vi "SubPanel_DataCollection_Rev11_v7.vi"(0 "DCPowerInformationClusterArray_Input":T2(array[cluster]), 1 "VISAPowerInfoInputArray":T7(array[cluster]), 2 "Run Data SubPanel Input":T6, 3 "RF Block Parameters":T5, 4 "Oscilloscope Info Array":T4(array[cluster]) {"vertical coupling" items=["AC", "DC", "Ground"]}, 6 "New Run?":bool, 7 "error in":errorcluster) -> (16 "data going into the binary file":T1, 20 "DCPowerInformationClusterArray_Output":T2(array[cluster]), 21 "VISAPowerInfoInputOutput":T7(array[cluster]), 22 "Run Data SubPanel Output":T6, 23 "RF Block Parameters Output":T5, 24 "Oscilloscope Info Array Output":T4(array[cluster]) {"vertical coupling" items=["AC", "DC", "Ground"]}, 25 "Reinitialize?":bool, 26 "Data Was Collected?":bool, 27 "error out":errorcluster)   [LabVIEW 2019]
uses:
  Controls/QueueDataControl.ctl
  Controls/DataBlockControl.ctl
  Controls/QueueDataControl_V2.ctl
  <vilib>/Analysis/NI_AALBase.lvlib
  Controls/QueueDataControl_V3.ctl
  <vilib>/Analysis/1siggen.llb/Ramp Pattern by Delta.vi
  <vilib>/Utility/file.llb/Write Delimited Spreadsheet (string).vi
  Controls/RFBlockControl.ctl
  <instrlib>/niScope/Controls/niScope vertical coupling.ctl
panel:
  out "Current 3":waveform(dbl)[](graph)
  out "Voltage 3":waveform(dbl)[](graph)
  out "DCPowerInfoArray":string[][](array[string])
  out "Array":string[][][](array[string])
  out "Current Measurements":cluster{dbl[], dbl[]}[](graph)
  out "Voltage Measurements":cluster{dbl[], dbl[]}[](graph)
  out "DCPowerInformationClusterArray_Input 2":T2(array[cluster])
  out "Exiting":bool
  out "Full Run Information":string
  out "Ready For Next Run?":bool
  in  "Next Run":bool
  out "Latchup Output Data":dbl[][](array[numeric])
  out "Recording Data":bool
  out "Current 2":waveform(dbl)[](graph)
  out "Voltage 2":waveform(dbl)[](graph)
  out "Current":waveform(dbl)[](graph)
  out "Voltage":waveform(dbl)[](graph)
  in  "End Collecting":bool
  in  "Record Data Toggle":bool
  out "error of collection":errorcluster
  in  "force exit SubVI":bool
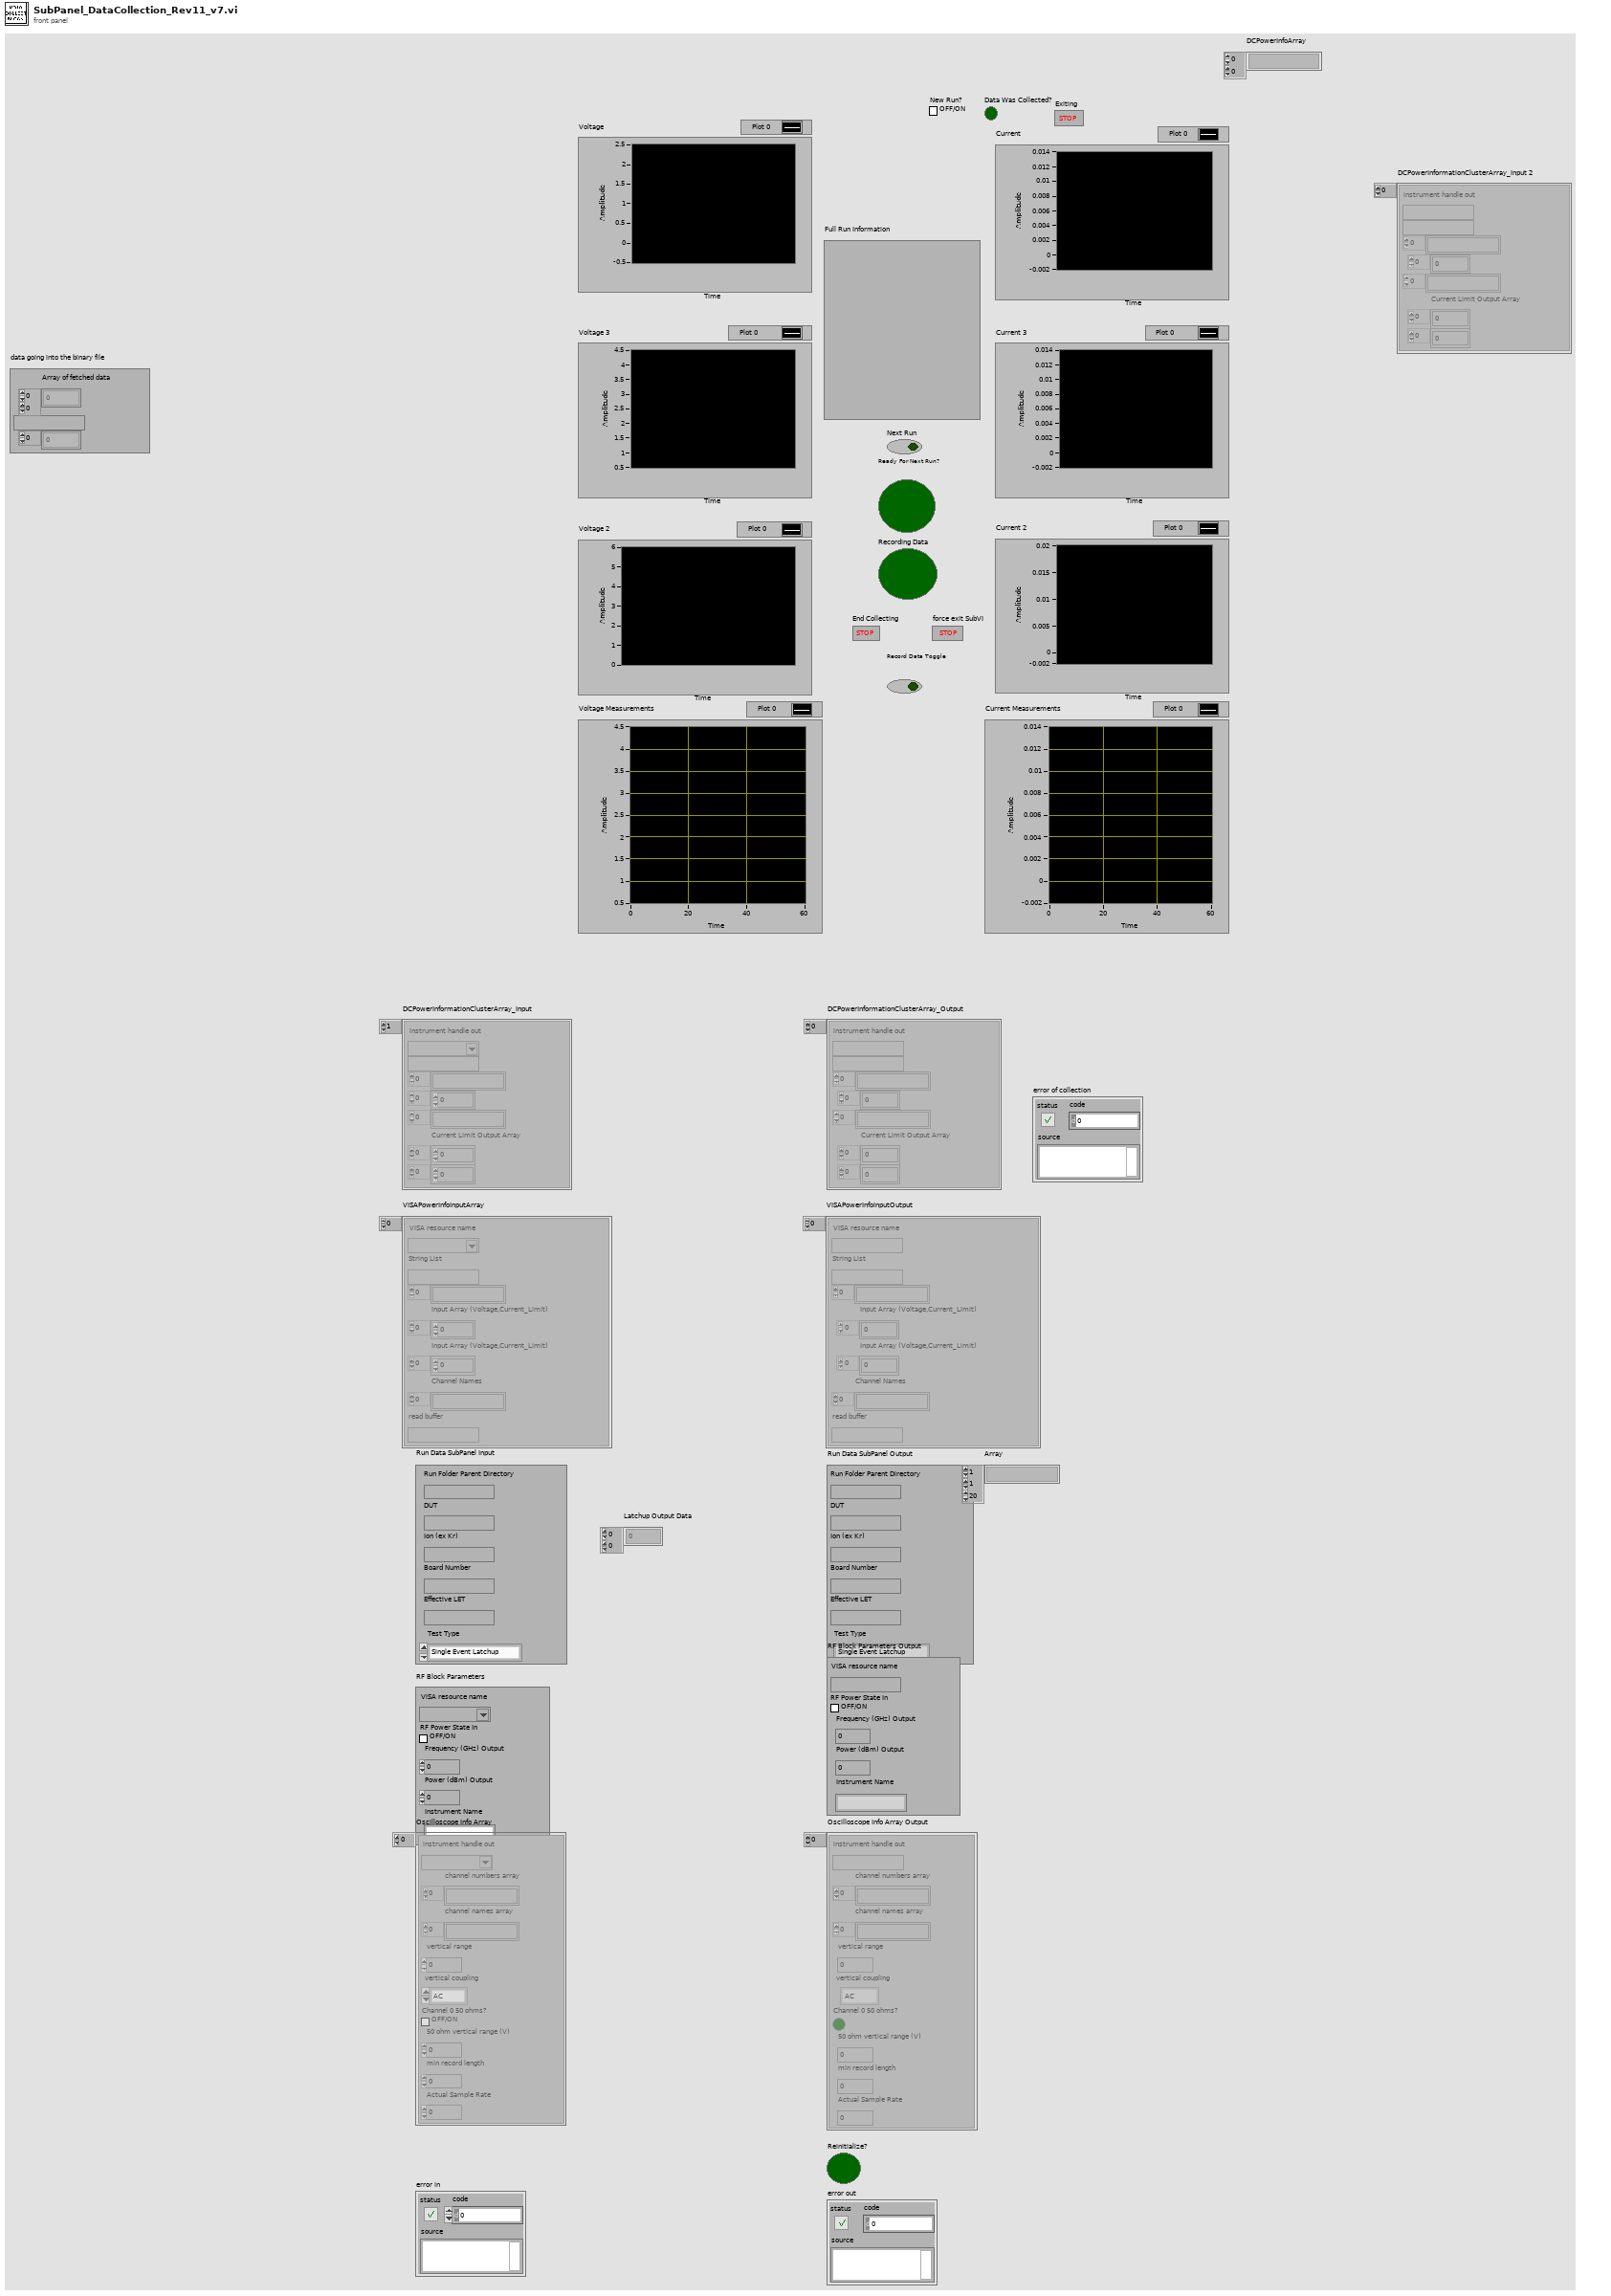
[diagram p1: front panel]
types:
  T1 = cluster{"Array of fetched data":dbl[][], string, i32[]}
  T2 = cluster{"instrument handle out":refnum<k15>, string, string[], dbl[], string[], "Current Limit Output Array":dbl[], dbl[]}[]
  T3 = typedef "niScope vertical coupling.ctl" = i32
  T4 = cluster{"instrument handle out":refnum<k15>, "channel numbers array":string[], "channel names array":string[], "vertical range":dbl, "vertical coupling":T3, "Channel 0 50 ohms?":bool, "50 ohm vertical range (V)":dbl, "min record length":i32, "Actual Sample Rate":dbl}[]
  T5 = typedef "RFBlockControl.ctl" = cluster{"VISA resource name":refnum<visa-resource-name>, "RF Power State In":bool, "Frequency (GHz) Output":dbl, "Power (dBm) Output":dbl, "Instrument Name":string}
  T6 = typedef "DataBlockControl.ctl" = cluster{"Run Folder Parent Directory":path, "DUT":string, "Ion (ex Kr)":string, "Board Number":string, "Effective LET":string, "Test Type":enum16{"Single Event Latchup", "Single Event Transient", "Single Event Upset"}}
  T7 = cluster{"VISA resource name":refnum<visa-resource-name>, "String List":string, string[], "Input Array (Voltage,Current_Limit)":dbl[], "Input Array (Voltage,Current_Limit)":dbl[], "Channel Names":string[], "read buffer":string}[]
  T8 = typedef "QueueDataControl_V3.ctl" = cluster{"Array of fetched data":dbl[][][], "Channel Names Array":string[], "Voltage Waveform Array":waveform(dbl)[], "Current Waveform Array":waveform(dbl)[], "Resetting Time":timestamp}
  T9 = typedef "QueueDataControl_V2.ctl" = cluster{"Time Stamp Array":timestamp[], "Initial Time":timestamp, "dt measurement array":dbl[], "samples per capture":i32[], "voltage measurements":dbl[][], "current measurements":dbl[][]}
  T10 = cluster{"IVI Refnum out":refnum<k15>, string, "voltage level channel 23":dbl, "Channel Name 23":string, "Current Limit":dbl, "Measure Record dt":dbl, string}[]
  T11 = cluster{"created path":path, "DCPowerInformation_byChannel":cluster{"IVI Refnum out":refnum<k15>, string, "voltage level channel 23":dbl, "Channel Name 23":string, "Current Limit":dbl, "Measure Record dt":dbl, string}[], string[]}
  T12 = typedef "QueueDataControl.ctl" = cluster{"Rolling Timer":timestamp, "Initial Time":timestamp, "dt between samples":dbl[], "number of samples per fetch":i32[], "voltage measurements":dbl[][], "current measurements":dbl[][]}
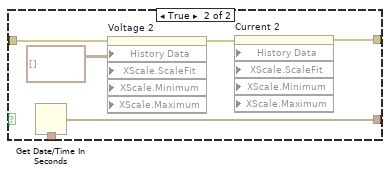
[diagram p2: hidden frame]
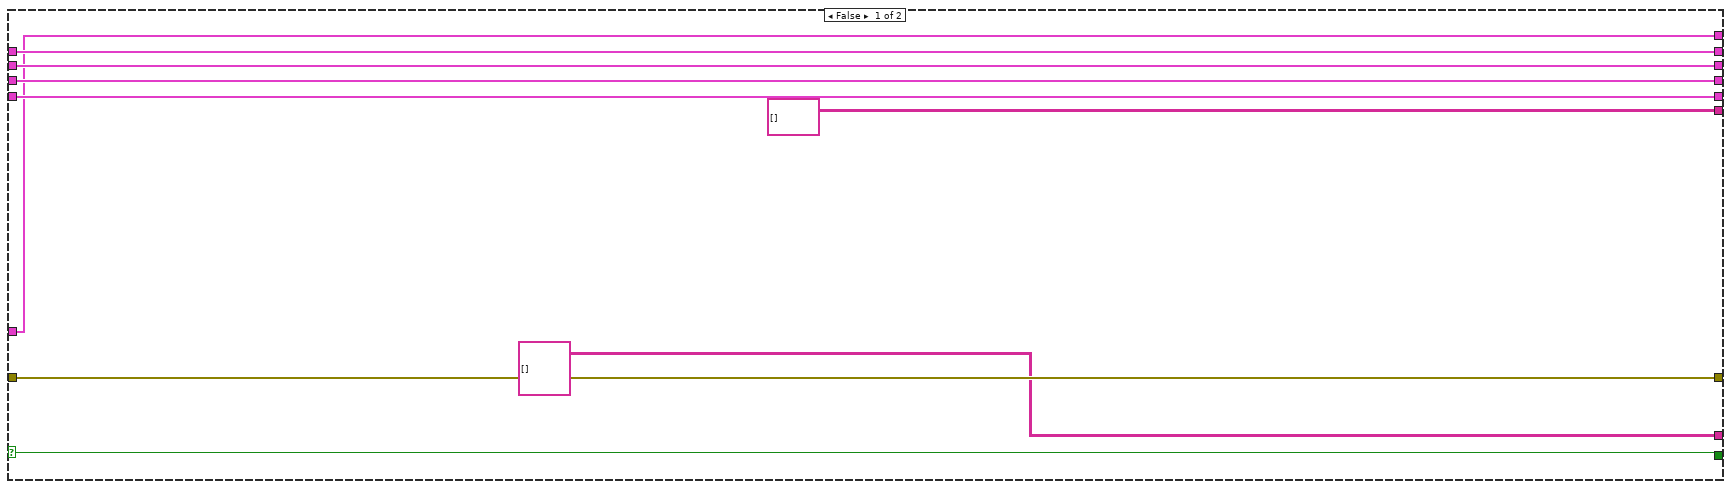
[diagram p4: hidden frame]
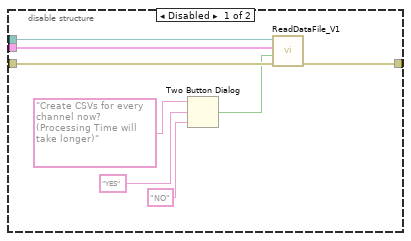
[diagram p5: hidden frame]
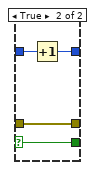
[diagram p6: hidden frame]
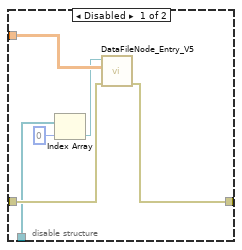
[diagram p9: hidden frame]
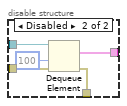
[diagram p10: hidden frame]
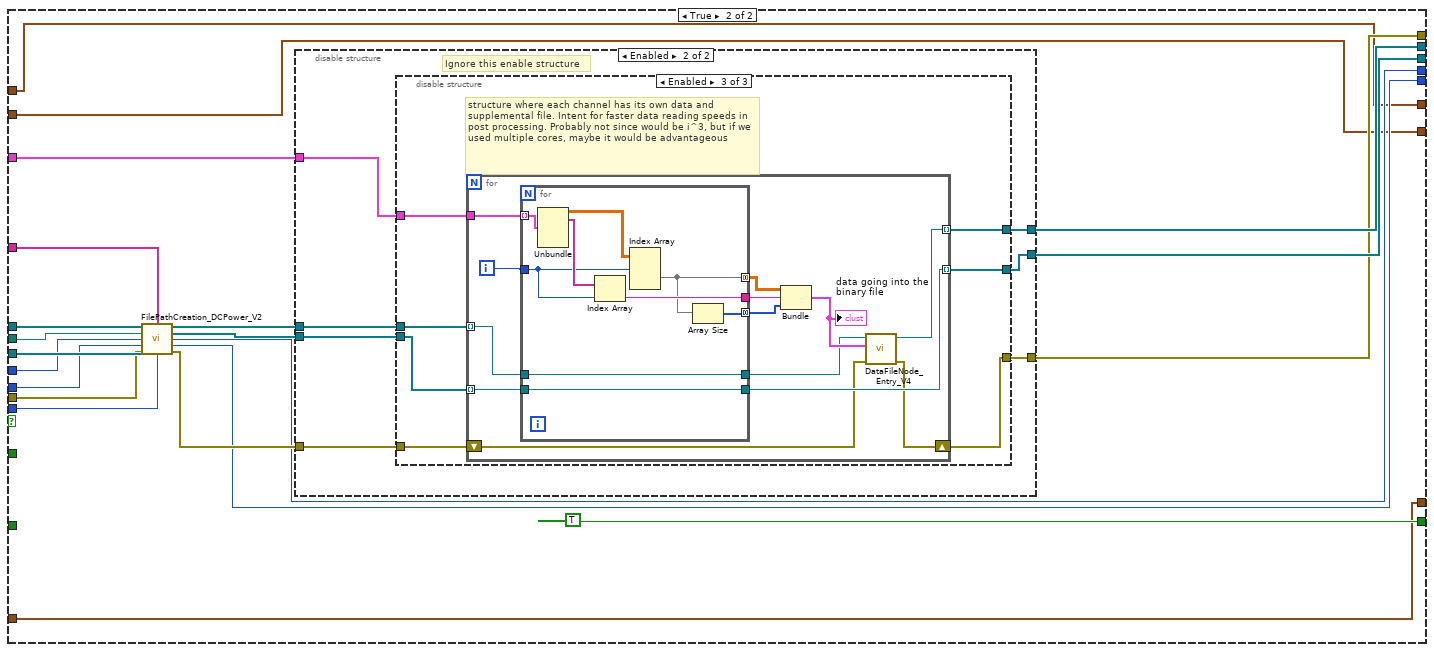
[diagram p13: hidden frame]
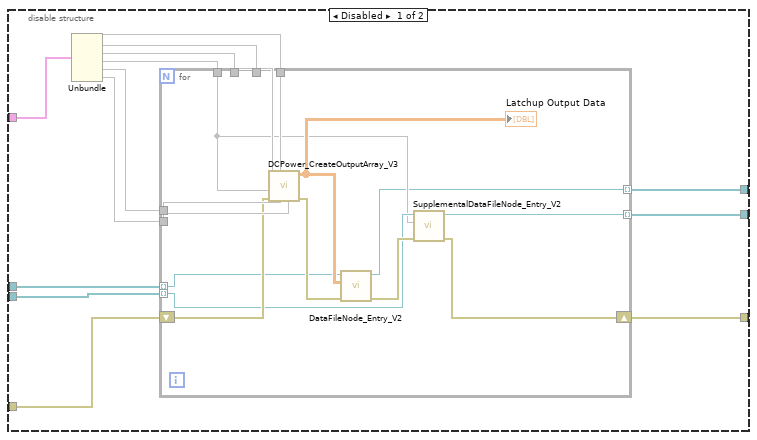
[diagram p14: hidden frame]
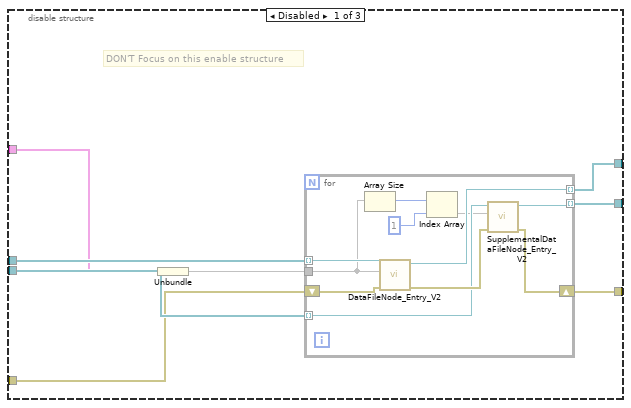
[diagram p15: hidden frame]
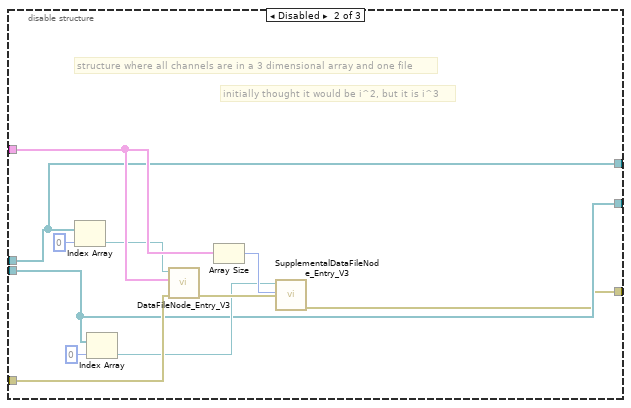
[diagram p16: hidden frame]
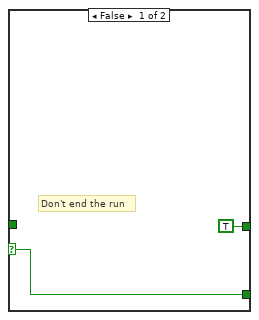
[diagram p18: hidden frame]
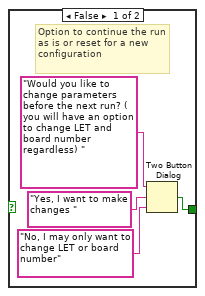
[diagram p19: hidden frame]
diagram:
  (unwired) string[] ["Instrument Name", "Channel Name", "Instrument Channel Number", "Voltage (V)", "Current Limit (A)", "Measure Record delta Time (s)"] ("new element/subarray")
  w53 = T8 {"Array of fetched data"=[], "Channel Names Array"=[], "Voltage Waveform Array"=[], "Current Waveform Array"=[], "Resetting Time"=timestamp(0 s since 1904-01-01)} ("DCPower Queue Data Double Array Format")
  (unwired) 10000 ("binary file indexor in")
  (unwired) T9 {"Time Stamp Array"=[], "Initial Time"=timestamp(0 s since 1904-01-01), "dt measurement array"=[], "samples per capture"=[], "voltage measurements"=[], "current measurements"=[]} ("DCPowerDataQueueControl_V2")
  (unwired) T6 {"Run Folder Parent Directory"=path "", "DUT"="", "Ion (ex Kr)"="", "Board Number"="", "Effective LET"="", "Test Type"=enum."Single Event Latchup"} ("Run Data Configuration")
  # "Reset the graph that is saving every 10 seconds of data. Every reset the low bound of the ten seconds is"
  # "Need to change to reflect number of channels that are being recorded. Collect this from a parameters file eventually that will be created"
  # "I don't think we are using these so we can just have them here for now. May need to include them later though"
  # "Indicator if the system is ready for another run. Also indicates if data was actually collected"
  # "Resets the system to start recording"
  # "A flag to ensure the warning message shows only once and doesn't lock the system"
  # "If I am going to reset the entire configuration or if we are going up in LET only. True, reset the system. False, don't reset the system"
  # "MAKE INTO SUBVI"
  n1 = flat-sequence {
    tunnel: [w96] -> w70
    tunnel: "error in" -> [w95]
    tunnel: [w100] -> w78
    tunnel: "Run Data SubPanel Input" -> [w93]
    frame #0 {
      n2 = local write "Recording Data"(FALSE ("Recording Data")) -> ()
      n3 = local write "Exiting"(FALSE ("Forced Exit")) -> ()
      n4 = call "Convert_RunInfoCluster_2_RunInfoStringList.vi"("error in"=w95, "Run Data SubPanel Input"=w93) -> ("error output"=w94:errorcluster, "Run Data Output"=w92:string)
      n5 = call "Display Message to User"("error in (no error)"=w94, "Enable"=TRUE, "Message"=w92) -> ("error out"=w96:errorcluster)  [unwired: 7 in, 1 out]
      n6 = Two Button Dialog(message="Changing the LET?", 1:"No" ("F button name (\"Cancel\")"), 2:"Yes" ("T button name (\"OK\")")) -> (T button?=w100:bool)
    }
  }
  n7 = call "Convert_InstrumentReferenceArray_2_ChannelReferenceArray.vi"("error in (no error)"=w70, "DCPowerInformationClusterArray_Input"="DCPowerInformationClusterArray_Input") -> ("error out"=w69:errorcluster, "DCPowerInformation_byChannel"=w23:T10)
  n8 = case shown="True" w78 {
    tunnel: "Run Data SubPanel Input" -> [w102 w106]
    tunnel: [w102 w105] -> w75
    tunnel: [w101 w104] -> w72
    tunnel: w69 -> [w101 w103]
    frame False {
    }
    frame True {
      n9 = call "Change_RunInfo.vi"("error in (no error)"=w103, "Run Data SubPanel in"=w106) -> ("error out"=w104:errorcluster, "Run Data SubPanel out"=w105:T6)
    }
  }
  n10 = Unbundle(w75) -> ("Run Folder Parent Directory"=w73:path)  [unwired: 5 out]
  n11 = List Folder(path=w73, error in=w72) -> (folder names=w74:string[], error out=w57:errorcluster)  [unwired: 2 in, 2 out]
  n12 = Array Size(array=w74) -> (size(s)=w60:i32)
  n13 = case shown="False" "New Run?" {
    selector: "New Run?" -> [w108 w111]
    tunnel: [w109 w113] -> w61
    tunnel: w60 -> [w109 w112]
    tunnel: [w108 w111] -> w59
    tunnel: [w107 w110] -> w58
    tunnel: w57 -> [w107 w110]
    frame False {
    }
    frame True {
      n14 = Increment(x=w112) -> (x+1=w113:i32)
    }
  }
  n15 = Number To Decimal String(number=w61) -> (decimal integer string=w64:string)  [unwired: 1 in]
  n16 = Concatenate Strings("Run_", w64) -> (w71:string)
  n17 = Array Size(array=w23) -> (size(s)=w56:i32)
  n18 = call "InitialFileFolderCreation_V2.vi"("New Run?"=w59, "error in (no error)"=w58, "Run Number"=w71, "DCPowerArrayClusterSize"=w56, "base path"=w73) -> ("error out"=w55:errorcluster, "SupplementalDataFileReferenceObjectArray"=w67:refnum<file>[], "DataFileReferenceObjectArray"=w68:refnum<file>[], "created path"=w6:path)  [unwired: 3 in]
  n19 = call "Convert_RunInfoCluster_2_RunInfoStringList.vi"("error in"=w55, "Run Data SubPanel Input"=w75) -> ("error output"=w4:errorcluster, "Run Data Output"=→"Full Run Information":string)
  n20 = for {
    shift-right: [w114] -> w3
    shift-left: w4 -> [w116]
    tunnel: "DCPowerInformationClusterArray_Input" -> [w118] mode=indexing
    n21 = Unbundle(w118) -> ("instrument handle out"=w115:refnum<k15>, w117:string)  [unwired: 5 out]
    n22 = call <instrlib>:"niDCPower Initiate With Channels.vi"("error in (no error)"=w116, "channel name"=w117, "instrument handle"=w115) -> ("error out"=w114:errorcluster)  [unwired: 7 in, 1 out]
  }
  n23 = disable-structure shown="Enabled" {
    disable-tunnel: w3 -> [w122 w124]
    disable-tunnel: [w121 w124] -> w83
    disable-tunnel: [w120 _] -> w84
    disable-tunnel: w53 -> [w119 _]
    frame Enabled {
      n24 = Obtain Queue(name (unnamed)="DCPowerQueue", element data type=w119, error in (no error)=w122) -> (queue out=w120:refnum<queue>, error out=w121:errorcluster)  [unwired: 2 in, 1 out]
    }
    frame Disabled {
    }
  }
  n25 = for {
    tunnel: w23 -> [w126] mode=indexing
    tunnel: [w125] -> w24 mode=indexing
    # "Creating Array of Channel Names"
    n26 = Unbundle(w126) -> ("Channel Name 23"=w125:string)  [unwired: 6 out]
  }
  n27 = Array Size(array=w24) -> (size(s)=w46:i32)
  n28 = Get Date/Time In Seconds() -> (seconds since 1Jan1904=w1:timestamp)
  n29 = Bundle("created path"=w6, "DCPowerInformation_byChannel"=w23, w24) -> (w22:T11)  [unwired: 1 in]
  n30 = disable-structure shown="Enabled" {
    disable-tunnel: "DCPowerInformationClusterArray_Input" -> [w136 _]
    disable-tunnel: "VISAPowerInfoInputArray" -> [_ _]
    disable-tunnel: w75 -> [_ _]
    disable-tunnel: "RF Block Parameters" -> [_ _]
    disable-tunnel: "Oscilloscope Info Array" -> [_ _]
    disable-tunnel: w84 -> [w145 _]
    disable-tunnel: w83 -> [w144 _]
    disable-tunnel: w24 -> [w143 _]
    disable-tunnel: w6 -> [w142 _]
    disable-tunnel: w68 -> [w141 _]
    disable-tunnel: w67 -> [w140 _]
    disable-tunnel: 0 ("binary file indexor in") -> [w139 _]
    disable-tunnel: 0 ("binary file indexor in") -> [w138 _]
    disable-tunnel: 1000 ("binary file indexor in") -> [w137 _]
    disable-tunnel: [w133 _] -> w50
    disable-tunnel: [w132 _] -> w52
    disable-tunnel: [w135 _] -> w51
    disable-tunnel: dbl[][][] [] -> [_ _]
    disable-tunnel: w46 -> [w131 _]
    disable-tunnel: FALSE -> [w130 _]
    frame Enabled {
      n31 = Get Date/Time In Seconds() -> (seconds since 1Jan1904=w127:timestamp)
      n32 = while {
        tunnel: w145 -> [w185]
        shift-right: [w172] -> w134
        shift-left: w144 -> [w184]
        tunnel: w142 -> [w181]
        shift-right: [w174] -> w132
        shift-left: w141 -> [w182]
        shift-right: [w173] -> w135
        shift-left: w140 -> [w180]
        shift-right: [w176] -> _
        shift-left: w139 -> [w179]
        shift-right: [w175] -> _
        shift-left: w138 -> [w178]
        tunnel: w137 -> [w177]
        tunnel: w143 -> [w183]
        tunnel: w131 -> [_]
        shift-right: [w161] -> _
        shift-left: w130 -> [w160]
        shift-right: [w157] -> _
        shift-left: waveform(dbl)[] [] ("array") -> [w158]
        shift-right: [w155] -> _
        shift-left: waveform(dbl)[] [] ("array") -> [w156]
        shift-right: [w153] -> _
        shift-left: w127 -> [w154]
        stop <- w169 stop-if-true
        # "If recording data is on, there should always be elements in the queue, so I shouldn't have to worry about a state where the \"recording data\" is active but there is no data in the queue, if so, then I'll just have to find an alternative to the OR statement"
        n33 = Get Queue Status(queue=w185, error in (no error)=w184) -> (queue out=w166:refnum<queue>, error out=w167:errorcluster, # elements in queue=w162:i32)  [unwired: 1 in, 5 out]
        n34 = disable-structure shown="Enabled" {
          disable-tunnel: [w189 w191] -> w168
          disable-tunnel: w167 -> [w188 w193]
          disable-tunnel: w166 -> [w187 w194]
          disable-tunnel: [w186 w190] -> w165
          frame Enabled {
            n35 = Flush Queue(queue=w187, error in (no error)=w188) -> (remaining elements=w186:T8[], error out=w189:errorcluster)  [unwired: 1 out]
          }
          frame Disabled {
            n36 = Dequeue Element(queue=w194, timeout in ms (-1)=100, error in (no error)=w193) -> (element=w190:T8, error out=w191:errorcluster)  [unwired: 2 out]
          }
        }
        n37 = Not Equal To 0?(x=w162) -> (x != 0?=w164:bool)
        n38 = And(x=w164, y="Record Data Toggle") -> (x .and. y?=w163:bool)
        n39 = case shown="False" w163 {
          tunnel: w165 -> [w200 w274]
          tunnel: w168 -> [w214 w268]
          tunnel: w183 -> [w215 w260]
          tunnel: w182 -> [w222 w273]
          tunnel: w181 -> [w216 w272]
          tunnel: w180 -> [w223 w271]
          tunnel: w179 -> [w221 w270]
          tunnel: w178 -> [w220 w259]
          tunnel: w177 -> [_ w258]
          tunnel: [w221 w267] -> w176
          tunnel: [w220 w266] -> w175
          tunnel: [w222 w263] -> w174
          tunnel: [w223 w262] -> w173
          tunnel: [w197 w261] -> w172
          tunnel: [w213 TRUE] -> w161
          tunnel: w160 -> [w212 _]
          tunnel: "Record Data Toggle" -> [w219 _]
          tunnel: w158 -> [w210 w256]
          tunnel: [w196 w256] -> w157
          tunnel: w156 -> [w209 w255]
          tunnel: [w195 w255] -> w155
          tunnel: w154 -> [w201 w254]
          tunnel: [w202 w254] -> w153
          frame False {
            n40 = Not(x=w219) -> (.not. x?=w218:bool)
            n41 = And(x=w218, y=w212) -> (x .and. y?=w217:bool)
            n42 = case shown="True" w217 {
              tunnel: w216 -> [_ w253]
              tunnel: w215 -> [_ w252]
              tunnel: w214 -> [w245 w250]
              tunnel: [w245 w249] -> w211
              tunnel: [w244 FALSE] -> w213
              tunnel: w212 -> [w244 _]
              frame False {
              }
              frame True {
                n43 = call "ReadDataFile_V1.vi"("error in (no error)"=w250, "Create CSV files?"=FALSE, "Channel Names Array"=w252, "DataFolder Path"=w253) -> ("error out"=w249:errorcluster, "Current Measurements"=→"Current Measurements":cluster{dbl[], dbl[]}[], "Voltage Measurements"=→"Voltage Measurements":cluster{dbl[], dbl[]}[])  [unwired: 5 in]
              }
            }
            n44 = Array Size(array=w200) -> (size(s)=w199:i32)
            n45 = for {
              shift-right: [w243] -> w198
              shift-left: w211 -> [w243]
              tunnel: w200 -> [w242] mode=indexing
              tunnel: w210 -> [w239]
              tunnel: [w236] -> w196
              tunnel: w209 -> [w238]
              tunnel: [w235] -> w195
              tunnel: [w237] -> w204
              tunnel: [w234] -> _
              tunnel: [w233] -> _
              tunnel: w199 -> [_]
              n46 = Unbundle(w242) -> ("Voltage Waveform Array"=w241:waveform(dbl)[], "Current Waveform Array"=w240:waveform(dbl)[], "Resetting Time"=w237:timestamp)  [unwired: 2 out]
              n47 = Insert Into Array(array=w239, new element=w241) -> (w236:waveform(dbl)[])  [unwired: 1 in]
              n48 = Insert Into Array(array=w238, new element=w240) -> (w235:waveform(dbl)[])  [unwired: 1 in]
              n49 = Array Size(array=w235) -> (size(s)=w234:i32)
              n50 = Array Size(array=w236) -> (size(s)=w233:i32)
            }
            n51 = To Double Precision Float(number=w204) -> (double precision float=w206:dbl)
            n52 = To Double Precision Float(number=w201) -> (double precision float=w205:dbl)
            n53 = Subtract(x=w206, y=w205) -> (x-y=w203:dbl)
            n54 = Greater?(x=w203, y=2.0) -> (0:w207:bool)
            n55 = case shown="True" w207 {
              tunnel: [w225 w228] -> w202
              tunnel: w201 -> [w225 _]
              tunnel: w198 -> [w224 w232]
              tunnel: [w224 w230] -> w197
              frame False {
              }
              frame True {
                (unwired) u8 0 ("X Scale.Scale Fit")
                w229 = waveform(dbl)[][] [] ("History Data")
                n56 = Get Date/Time In Seconds() -> (seconds since 1Jan1904=w228:timestamp)
                n57 = To Double Precision Float(number=w228) -> (double precision float=w226:dbl)
                n58 = Add(x=w226, y=2.0) -> ()  [unwired: 1 out]
                n59 = property on="Voltage 3" class="WFChart (strict)"(error in=w232, "History Data"=w229) -> (error out=w231:errorcluster)  [unwired: 1 in, 1 out]
                n60 = property on="Current 3" class="WFChart (strict)"(error in=w231, "History Data"=w229) -> (error out=w230:errorcluster)  [unwired: 1 in, 1 out]
              }
            }
          }
          frame True {
            n61 = call "FilePathCreation_DCPower_V2.vi"("binary file input reference array 1"=w273, "Channel Name Input array"=w260, "data output directory folder"=w272, "binary file indexor in"=w270, "Reset counter in"=w259, "error in (no error)"=w268, "binary file input reference array 2"=w271, "reset threshold"=w258) -> ("binary file output reference array"=w265:refnum<file>[], "binary file output reference array 2"=w264:refnum<file>[], "binary file indexor out"=w267:i32, "reset counter out"=w266:i32, "error out"=w269:errorcluster)  [unwired: 3 in]
            n62 = disable-structure shown="Enabled" {
              disable-tunnel: w274 -> [w287 w303]
              disable-tunnel: w269 -> [w286 w307]
              disable-tunnel: w265 -> [w285 w309]
              disable-tunnel: w264 -> [w284 w308]
              disable-tunnel: [w283 w306] -> w263
              disable-tunnel: [w282 w305] -> w262
              disable-tunnel: [w281 w304] -> w261
              frame Disabled {
                n63 = Unbundle(w287) -> (w275, w276, w280, w279, w278, w277)
                n64 = for {
                  tunnel: w280 -> [w300]
                  tunnel: w279 -> [w290]
                  tunnel: w278 -> [w299]
                  tunnel: w277 -> [w298]
                  tunnel: w276 -> [w301]
                  tunnel: w275 -> [w302]
                  shift-right: [w292] -> w281
                  shift-left: w286 -> [w297]
                  tunnel: w285 -> [w294] mode=indexing
                  tunnel: w284 -> [w291] mode=indexing
                  tunnel: [w289] -> w283 mode=indexing
                  tunnel: [w288] -> w282 mode=indexing
                  n65 = call "DCPower_CreateOutputArray_V3.vi"("current measurements"=w298, "voltage measurements"=w299, "Time Stamp Array"=w302, "error in"=w297, "actual count"=w290, "Measure Record dt"=w300, "Initial Time"=w301) -> ("error out"=w296:errorcluster, "Data Output Array"=w295:dbl[][])  [unwired: 3 in]
                  "Latchup Output Data" <- w295
                  n66 = call "DataFileNode_Entry_V2.vi"("error in (no error)"=w296, "Data Output Array"=w295, "Byte Stream File in"=w294) -> ("error out"=w293:errorcluster, "Byte Stream File out"=w289:refnum<file>)  [unwired: 7 in]
                  n67 = call "SupplementalDataFileNode_Entry_V2.vi"("error in (no error)"=w293, "actual count"=w290, "Byte Stream File in"=w291) -> ("error out"=w292:errorcluster, "Byte Stream File out"=w288:refnum<file>)  [unwired: 7 in]
                }
              }
              frame Enabled {
                # "Ignore this enable structure"
                n68 = disable-structure shown="Enabled" {
                  disable-tunnel: w309 -> [w317 w331 w342]
                  disable-tunnel: w308 -> [w316 w330 w343]
                  disable-tunnel: w307 -> [w315 w339 w345]
                  disable-tunnel: [w314 w331 w340] -> w306
                  disable-tunnel: [w313 w330 w341] -> w305
                  disable-tunnel: [w312 w329 w346] -> w304
                  disable-tunnel: w303 -> [w311 w336 w344]
                  frame Disabled {
                    # "DON'T Focus on this enable structure"
                    n69 = Unbundle(w311) -> (w310)
                    n70 = for {
                      tunnel: w310 -> [w325]
                      tunnel: w317 -> [w327] mode=indexing
                      tunnel: w316 -> [w326] mode=indexing
                      tunnel: [w323] -> w314 mode=indexing
                      tunnel: [w322] -> w313 mode=indexing
                      shift-right: [w321] -> w312
                      shift-left: w315 -> [w324]
                      n71 = Array Size(array=w325) -> (size(s)=w320:i32)
                      n72 = call "DataFileNode_Entry_V2.vi"("error in (no error)"=w324, "Data Output Array"=w325, "Byte Stream File in"=w327) -> ("error out"=w328:errorcluster, "Byte Stream File out"=w323:refnum<file>)  [unwired: 7 in]
                      n73 = Index Array(array=w320, index=1) -> (element=w318)
                      n74 = call "SupplementalDataFileNode_Entry_V2.vi"("error in (no error)"=w328, "actual count"=w318, "Byte Stream File in"=w326) -> ("error out"=w321:errorcluster, "Byte Stream File out"=w322:refnum<file>)  [unwired: 7 in]
                    }
                  }
                  frame Disabled {
                    # "initially thought it would be i^2, but it is i^3"
                    # "structure where all channels are in a 3 dimensional array and one file"
                    n75 = Index Array(array=w331, index=0) -> (element=w332:refnum<file>)
                    n76 = Index Array(array=w330, index=0) -> (element=w333:refnum<file>)
                    n77 = call "DataFileNode_Entry_V3.vi"("error in (no error)"=w339, "remaining elements"=w336, "Byte Stream File in"=w332) -> ("error out"=w338:errorcluster)  [unwired: 7 in, 1 out]
                    n78 = Array Size(array=w336) -> (size(s)=w337:i32)
                    n79 = call "SupplementalDataFileNode_Entry_V3.vi"("error in (no error)"=w338, "actual count"=w337, "Byte Stream File in"=w333) -> ("error out"=w329:errorcluster)  [unwired: 7 in, 1 out]
                  }
                  frame Enabled {
                    # "structure where each channel has its own data and supplemental file. Intent for faster data reading speeds in post processing. Probably not since would be i^3, but if we used multiple cores, maybe it would be advantageous"
                    n80 = for {
                      shift-right: [w348] -> w346
                      shift-left: w345 -> [w349]
                      tunnel: w344 -> [w359]
                      tunnel: w343 -> [w356] mode=indexing
                      tunnel: w342 -> [w355] mode=indexing
                      tunnel: [w354] -> w341 mode=indexing
                      tunnel: [w347] -> w340 mode=indexing
                      i -> [w353]
                      n81 = for {
                        tunnel: w359 -> [w368] mode=indexing
                        tunnel: w353 -> [w365]
                        tunnel: [w361] -> w352 mode=concatenating
                        tunnel: [w364] -> w358
                        tunnel: w356 -> [w362]
                        tunnel: w355 -> [w363]
                        tunnel: [w363] -> w350
                        tunnel: [w362] -> w354
                        tunnel: [w360] -> w357 mode=concatenating
                        n82 = Unbundle(w368) -> ("Array of fetched data"=w367:dbl[][][], "Channel Names Array"=w366:string[])  [unwired: 3 out]
                        n83 = Index Array(array=w366, index=w365) -> (element=w364:string)
                        n84 = Index Array(array=w367, index (dim 0)=w365) -> (element=w361:dbl[][])  [unwired: 2 in]
                        n85 = Array Size(array=w361) -> (size(s)=w360:i32[])
                      }
                      n86 = Bundle("Array of fetched data"=w352, w358, w357) -> (w351:T1)  [unwired: 1 in]
                      "data going into the binary file" <- w351
                      n87 = call "DataFileNode_Entry_V4.vi"("error in (no error)"=w349, "Queued Elements"=w351, "Byte Stream File in"=w350) -> ("error out"=w348:errorcluster, "Byte Stream File out"=w347:refnum<file>)  [unwired: 7 in]
                    }
                  }
                }
              }
            }
          }
        }
        "Voltage 3" <- w157
        "Current 3" <- w155
        n88 = local read "Exiting"() -> (w171:bool)
        n89 = Equal To 0?(x=w162) -> (x = 0?=w170:bool)
        n90 = And(x=w170, y=w171) -> (x .and. y?=w169:bool)
      }
      n91 = disable-structure shown="Enabled" {
        disable-tunnel: _ -> [w151 _]
        disable-tunnel: w134 -> [w150 w152]
        disable-tunnel: [w149 w152] -> w133
        disable-tunnel: w132 -> [w148 _]
        frame Disabled {
          n92 = Index Array(array=w148, index=0) -> (element=w146:refnum<file>)
          n93 = call "DataFileNode_Entry_V5.vi"("error in (no error)"=w150, "Data to be inputter"=w151, "Byte Stream File in"=w146) -> ("error out"=w149:errorcluster)  [unwired: 7 in, 1 out]
        }
        frame Enabled {
          (unwired) T1 {"Array of fetched data"=[], "", []} ("cluster")
        }
      }
      "DCPowerInformationClusterArray_Input 2" <- w136
    }
    frame Disabled {
    }
  }
  n94 = while {
    shift-right: [w402] -> w11
    shift-left: "DCPowerInformationClusterArray_Input" -> [w402]
    shift-right: [w406] -> w13
    shift-left: "VISAPowerInfoInputArray" -> [w406]
    shift-right: [w405] -> w15
    shift-left: w75 -> [w405]
    shift-right: [w404] -> w17
    shift-left: "RF Block Parameters" -> [w404]
    shift-right: [w403] -> w19
    shift-left: "Oscilloscope Info Array" -> [w403]
    shift-right: [w386] -> w54
    shift-left: _ -> [w399]
    tunnel: w23 -> [w401]
    tunnel: w23 -> [w400]
    shift-right: [w396] -> _
    shift-left: FALSE -> [w393]
    tunnel: w84 -> [w395]
    shift-right: [w376] -> _
    shift-left: FALSE -> [w381]
    tunnel: [w384] -> w82
    shift-right: [w379] -> _
    shift-left: TRUE ("x .and. y?") -> [w380]
    shift-right: [w377] -> _
    shift-left: w1 -> [w378]
    tunnel: [w376] -> w10
    tunnel: w24 -> [w374]
    tunnel: w53 -> [w373]
    shift-right: [w371] -> _
    shift-left: w1 -> [w372]
    stop <- w375 stop-if-true
    n95 = local read "Recording Data"() -> (w369:bool)
    n96 = Not(x=w381) -> (.not. x?=w382:bool)
    n97 = And(x=w369, y=w382) -> (x .and. y?=w383:bool)
    "Recording Data" <- w383
    n98 = Not(x=w383) -> (.not. x?=w394:bool)
    n99 = case shown="True" TRUE {
      tunnel: w399 -> [_ w534]
      tunnel: w401 -> [_ w533]
      tunnel: w400 -> [w436 w531]
      tunnel: w399 -> [w433 w529]
      tunnel: [w421 w515] -> w398
      tunnel: [w422 w516] -> w397
      tunnel: w393 -> [_ w526]
      tunnel: [FALSE w527] -> w396
      tunnel: w395 -> [_ w525]
      tunnel: [w434 w523] -> w391
      tunnel: w369 -> [w430 _]
      tunnel: w381 -> [w431 _]
      tunnel: w380 -> [w426 _]
      tunnel: [w427 TRUE] -> w379
      tunnel: w378 -> [w425 w530]
      tunnel: [w425 w522] -> w377
      tunnel: w374 -> [_ _]
      tunnel: w373 -> [_ w519]
      tunnel: w372 -> [w424 w517]
      tunnel: [w423 w517] -> w371
      frame False {
        n100 = And(x=w430, y=w431) -> (x .and. y?=w429:bool)
        n101 = And(x=w426, y=w429) -> (x .and. y?=w428:bool)
        n102 = case shown="True" w428 {
          tunnel: [w510 w512] -> w432
          tunnel: w433 -> [w510 w513]
          tunnel: [w509 FALSE] -> w427
          tunnel: w426 -> [w509 _]
          frame False {
          }
          frame True {
            n103 = call "Display Message to User2"("error in (no error)"=w513) -> ("error out"=w512:errorcluster)  [unwired: 9 in, 1 out]
          }
        }
        n104 = disable-structure shown="Enabled" {
          disable-tunnel: w436 -> [w446 w483]
          disable-tunnel: [w441 w482] -> w422
          disable-tunnel: [w440 w480] -> w421
          disable-tunnel: [w438 w470] -> w434
          disable-tunnel: w432 -> [w437 w481]
          disable-tunnel: w425 -> [_ _]
          disable-tunnel: w424 -> [_ w472]
          disable-tunnel: [_ w471] -> w423
          frame Disabled {
            n105 = call "Fetch&Process_Measurements.vi"("error in (no error)"=w437, "DCPowerInformation_byChannel"=w446) -> ("error out"=w447:errorcluster, "Current Measurement"=w440:waveform(dbl)[], "Voltage Measurement"=w441:waveform(dbl)[], "Rolling Timer Output"=w439:timestamp, "Rolling Timer Input"=w444:timestamp, "Queue Data Parameters in"=w445:T12)  [unwired: 3 in, 1 out]
            n106 = Subtract(x=w439, y=w442) -> (x-y=w449:dbl)
            n107 = Greater?(x=w449, y=10.0) -> (0:w448:bool)
            n108 = disable-structure shown="Enabled" {
              disable-tunnel: w448 -> [w456 _]
              disable-tunnel: w447 -> [w455 w469]
              disable-tunnel: [w454 w469] -> w438
              disable-tunnel: [w453 w468] -> w443
              disable-tunnel: w439 -> [w452 w468]
              disable-tunnel: [w451 _] -> w442
              frame Enabled {
                n109 = case shown="True" w456 {
                  tunnel: w455 -> [w458 w464]
                  tunnel: [w458 w462] -> w454
                  tunnel: [w457 w466] -> w453
                  tunnel: w452 -> [_ w466]
                  tunnel: w451 -> [w457 _]
                  frame False {
                  }
                  frame True {
                    w461 = u8 0 ("X Scale.Scale Fit")
                    w465 = waveform(dbl)[][] [] ("History Data")
                    n110 = To Double Precision Float(number=w466) -> (double precision float=w459:dbl)
                    n111 = Add(x=w459, y=10.0) -> (x+y=w460:dbl)
                    n112 = property on="Voltage 2" class="WFChart (strict)"(error in=w464, "History Data"=w465, "XScale.ScaleFit"=w461, "XScale.Minimum"=w459, "XScale.Maximum"=w460) -> (error out=w463:errorcluster)  [unwired: 1 in, 1 out]
                    n113 = property on="Current 2" class="WFChart (strict)"(error in=w463, "History Data"=w465, "XScale.ScaleFit"=w461, "XScale.Minimum"=w459, "XScale.Maximum"=w460) -> (error out=w462:errorcluster)  [unwired: 1 in, 1 out]
                  }
                }
              }
              frame Disabled {
              }
            }
          }
          frame Enabled {
            n114 = for {
              tunnel: w483 -> [w508] mode=indexing
              tunnel: [w501] -> w482 mode=indexing
              tunnel: [w500] -> w480 mode=indexing
              shift-right: [w497] -> w473
              shift-left: w481 -> [w505]
              tunnel: [w495] -> w477
              n115 = Unbundle(w508) -> ("IVI Refnum out"=w504:refnum<k15>, w507:string, "Measure Record dt"=w496:dbl)  [unwired: 4 out]
              n116 = property class="niDCPower"(reference=w504, error in=w505, "Active Channel"=w507) -> (reference out=w503:refnum<k15>, error out=w502:errorcluster, "Fetch Backlog"=w506:i32)
              n117 = Get Date/Time In Seconds() -> (seconds since 1Jan1904=w495:timestamp)
              n118 = call <instrlib>:"niDCPower Fetch Multiple.vi"("instrument handle"=w503, "channel name"=w507, "count (1)"=w506, "error in (no error)"=w502) -> ("voltage measurements"=w498:dbl[], "current measurements"=w499:dbl[], "error out"=w497:errorcluster)  [unwired: 6 in, 3 out]
              n119 = Bundle By Name("Y"=w499, "dt"=w496, "t0"=w495) -> (w500:waveform(dbl))  [unwired: 1 out]
              n120 = Bundle By Name("Y"=w498, "dt"=w496, "t0"=w495) -> (w501:waveform(dbl))  [unwired: 1 out]
            }
            n121 = To Double Precision Float(number=w477) -> (double precision float=w478:dbl)
            n122 = To Double Precision Float(number=w472) -> (double precision float=w479:dbl)
            n123 = Subtract(x=w478, y=w479) -> (x-y=w476:dbl)
            n124 = Greater?(x=w476, y=10.0) -> (0:w474:bool)
            n125 = case shown="True" w474 {
              tunnel: w473 -> [w484 w494]
              tunnel: [w485 w491] -> w471
              tunnel: w472 -> [w485 _]
              tunnel: [w484 w492] -> w470
              frame False {
              }
              frame True {
                w490 = u8 0 ("X Scale.Scale Fit")
                w489 = waveform(dbl)[][] [] ("History Data")
                n126 = Get Date/Time In Seconds() -> (seconds since 1Jan1904=w491:timestamp)
                n127 = To Double Precision Float(number=w491) -> (double precision float=w487:dbl)
                n128 = Add(x=10.0, y=w487) -> (x+y=w486:dbl)
                n129 = property on="Voltage 2" class="WFChart (strict)"(error in=w494, "History Data"=w489, "XScale.ScaleFit"=w490, "XScale.Minimum"=w487, "XScale.Maximum"=w486) -> (error out=w493:errorcluster)  [unwired: 1 in, 1 out]
                n130 = property on="Current 2" class="WFChart (strict)"(error in=w493, "History Data"=w489, "XScale.ScaleFit"=w490, "XScale.Minimum"=w487, "XScale.Maximum"=w486) -> (error out=w492:errorcluster)  [unwired: 1 in, 1 out]
              }
            }
          }
        }
      }
      frame True {
        (unwired) waveform(dbl)[] [] ("array")
        (unwired) waveform(dbl)[] []
        n131 = case shown="False" w526 {
          tunnel: [w567 w575] -> w522
          tunnel: w530 -> [_ w575]
          tunnel: w529 -> [w572 w574]
          tunnel: [w570 w574] -> w528
          tunnel: [TRUE w573] -> w527
          tunnel: w526 -> [_ w573]
          frame False {
            w563 = waveform(dbl)[][] [] ("History Data")
            w568 = u8 0 ("X Scale.Scale Fit")
            n132 = Get Date/Time In Seconds() -> (seconds since 1Jan1904=w567:timestamp)
            n133 = To Double Precision Float(number=w567) -> (double precision float=w564:dbl)
            n134 = Add(x=10.0 ("y"), y=w564) -> (x+y=w566:dbl)
            n135 = property on="Voltage 2" class="WFChart (strict)"(error in=w572, "History Data"=w563, "XScale.ScaleFit"=w568, "XScale.Minimum"=w564, "XScale.Maximum"=w566) -> (error out=w571:errorcluster)  [unwired: 1 in, 1 out]
            n136 = property on="Current 2" class="WFChart (strict)"(error in=w571, "History Data"=w563, "XScale.ScaleFit"=w568, "XScale.Minimum"=w564, "XScale.Maximum"=w566) -> (error out=w570:errorcluster)  [unwired: 1 in, 1 out]
          }
          frame True {
          }
        }
        n137 = for {
          tunnel: w531 -> [w562] mode=indexing
          tunnel: [w555] -> w516 mode=indexing
          tunnel: [w554] -> w515 mode=indexing
          shift-right: [w537] -> w524
          shift-left: w528 -> [w559]
          tunnel: w522 -> [w542]
          tunnel: [w541] -> w521 mode=indexing
          tunnel: [w540] -> w520 mode=indexing
          tunnel: [w535] -> w514
          n138 = Unbundle(w562) -> ("IVI Refnum out"=w558:refnum<k15>, w561:string, "Channel Name 23"=w540:string)  [unwired: 4 out]
          n139 = property class="niDCPower"(reference=w558, error in=w559, "Active Channel"=w561) -> (reference out=w557:refnum<k15>, error out=w556:errorcluster, "Fetch Backlog"=w560:i32)
          n140 = call <instrlib>:"niDCPower Fetch Multiple.vi"("instrument handle"=w557, "channel name"=w561, "count (1)"=w560, "error in (no error)"=w556) -> ("actual count"=w543:i32, "instrument handle out"=w539:refnum<k15>, "voltage measurements"=w545:dbl[], "current measurements"=w544:dbl[], "error out"=w538:errorcluster)  [unwired: 6 in, 1 out]
          n141 = property class="niDCPower"(reference=w539, error in=w538) -> (error out=w537:errorcluster, "Measure Record dt"=w536:dbl)  [unwired: 1 out]
          n142 = Get Date/Time In Seconds() -> (seconds since 1Jan1904=w535:timestamp)
          n143 = Bundle By Name("Y"=w545, "dt"=w536, "t0"=w535) -> (w555:waveform(dbl))  [unwired: 1 out]
          n144 = Bundle By Name("Y"=w544, "dt"=w536, "t0"=w535) -> (w554:waveform(dbl))  [unwired: 1 out]
          n145 = To Double Precision Float(number=w535) -> (double precision float=w551:dbl)
          n146 = To Double Precision Float(number=w542) -> (double precision float=w550:dbl)
          n147 = call-poly <vilib>:"Ramp Pattern.vi"("start"=1.0, "end"=w543, "delta"=1.0) -> ("Ramp Pattern"=w547:dbl[])  [unwired: 6 in, 2 out]
          n148 = Multiply(x=w536, y=w547) -> (x*y=w546:dbl[])
          n149 = Subtract(x=w551, y=w550) -> (x-y=w548:dbl)
          n150 = Add(x=w548, y=w546) -> (x+y=w553:dbl[])
          n151 = Build Array(w553, w545, w544) -> (w541:dbl[][])
        }
        n152 = disable-structure shown="Disabled" {
          disable-tunnel: w534 -> [w579 _]
          disable-tunnel: w533 -> [w578 _]
          disable-tunnel: [w577 errorcluster {"status"=FALSE, "code"=0, "source"=""} ("error out")] -> _
          frame Disabled {
            n153 = Get Date/Time In Seconds() -> (seconds since 1Jan1904=w576:timestamp)
            n154 = while {
              shift-right: [w583] -> w577
              shift-left: w579 -> [w594]
              tunnel: w578 -> [w595]
              tunnel: w576 -> [w591]
              shift-right: [w581] -> _
              shift-left: w576 -> [w592]
              tunnel: [w590] -> _
              shift-right: [w582] -> _
              shift-left: w576 -> [w580]
              stop <- "End Collecting" stop-if-true
              n155 = call "Fetch&Process_Measurements.vi"("Rolling Timer Input"=w592, "error in (no error)"=w594, "Initial Time"=w591, "DCPowerInformation_byChannel"=w595, "Queue Data Parameters in"=T12 {"Rolling Timer"=timestamp(0 s since 1904-01-01), "Initial Time"=timestamp(0 s since 1904-01-01), "dt between samples"=[], "number of samples per fetch"=[], "voltage measurements"=[], "current measurements"=[]} ("Queue Data Parameters")) -> ("error out"=w584:errorcluster, "Current Measurement"=→"Current":waveform(dbl)[], "Voltage Measurement"=→"Voltage":waveform(dbl)[], "Queue Data Parameters out"=w590:T12, "Rolling Timer Output"=w581:timestamp)  [unwired: 2 in]
              n156 = Subtract(x=w581, y=w580) -> (x-y=w586:dbl)
              n157 = Greater?(x=w586, y=10.0) -> (0:w585:bool)
              n158 = disable-structure shown="Enabled" {
                disable-tunnel: w585 -> [w602 _]
                disable-tunnel: w584 -> [w601 w615]
                disable-tunnel: [w600 w615] -> w583
                disable-tunnel: [w599 w614] -> w582
                disable-tunnel: w581 -> [w598 w614]
                disable-tunnel: w580 -> [w597 _]
                frame Enabled {
                  n159 = case shown="True" w602 {
                    tunnel: w601 -> [w604 w613]
                    tunnel: [w604 w611] -> w600
                    tunnel: [w603 w605] -> w599
                    tunnel: w598 -> [_ w605]
                    tunnel: w597 -> [w603 _]
                    frame False {
                    }
                    frame True {
                      w608 = u8 0 ("X Scale.Scale Fit")
                      w609 = waveform(dbl)[][] [] ("History Data")
                      n160 = To Double Precision Float(number=w605) -> (double precision float=w606:dbl)
                      n161 = Add(x=w606, y=10.0) -> (x+y=w607:dbl)
                      n162 = property on="Voltage" class="WFChart (strict)"(error in=w613, "History Data"=w609, "XScale.ScaleFit"=w608, "XScale.Minimum"=w606, "XScale.Maximum"=w607) -> (error out=w612:errorcluster)  [unwired: 1 in, 1 out]
                      n163 = property on="Current" class="WFChart (strict)"(error in=w612, "History Data"=w609, "XScale.ScaleFit"=w608, "XScale.Minimum"=w606, "XScale.Maximum"=w607) -> (error out=w611:errorcluster)  [unwired: 1 in, 1 out]
                    }
                  }
                }
                frame Disabled {
                }
              }
            }
          }
          frame Enabled {
          }
        }
        n164 = Bundle(cluster=w519, "Array of fetched data"=w521, "Channel Names Array"=w520, "Voltage Waveform Array"=w516, "Current Waveform Array"=w515, "Resetting Time"=w514) -> (w518:T8)
        n165 = Enqueue Element(queue=w525, element=w518, error in (no error)=w524) -> (error out=w523:errorcluster)  [unwired: 1 in, 2 out]
      }
    }
    "Voltage 2" <- w397
    "Current 2" <- w398
    n166 = And(x=w394, y=w393) -> (x .and. y?=w392:bool)
    n167 = case shown="True" w392 {
      tunnel: w391 -> [w417 w419]
      tunnel: [w418 TRUE] -> w376
      tunnel: w381 -> [w418 _]
      tunnel: [w417 w419] -> w386
      frame False {
      }
      frame True {
      }
    }
    "error of collection" <- w386
    "Ready For Next Run?" <- w376
    n168 = Or(x=w386, y="force exit SubVI") -> (x .or. y?=w388:bool)
    n169 = And(x="Next Run", y=w376) -> (x .and. y?=w390:bool)
    n170 = Or(x=w388, y=w390) -> (x .or. y?=w389:bool)
    n171 = case shown="True" w389 {
      selector: w389 -> [w408 _]
      tunnel: w388 -> [_ w411]
      tunnel: [w408 TRUE] -> w375
      tunnel: [TRUE ("T button?") w409] -> w384
      frame False {
        # "Don't end the run"
      }
      frame True {
        n172 = case shown="True" w411 {
          tunnel: [w412 TRUE] -> w409
          frame False {
            # "Option to continue the run as is or reset for a new configuration"
            n173 = Two Button Dialog(message="Would you like to change parameters before the next run? ( you will have an option to change LET and board number regardless) ", 1:"No, I may only want to change LET or board number" ("F button name (\"Cancel\")"), 2:"Yes, I want to make changes " ("T button name (\"OK\")")) -> (T button?=w412:bool)
          }
          frame True {
            # "End the run immediately. There is an error or an immediate issue with the VI"
          }
        }
      }
    }
    "Exiting" <- w375
  }
  "Reinitialize?" <- w82
  n174 = for {
    tunnel: w52 -> [w621] mode=indexing
    tunnel: w51 -> [w619] mode=indexing
    shift-right: [w617] -> w49
    shift-left: w50 -> [w620]
    n175 = Close File(refnum=w621, error in=w620) -> (error out=w618:errorcluster)  [unwired: 1 out]
    n176 = Close File(refnum=w619, error in=w618) -> (error out=w617:errorcluster)  [unwired: 1 out]
  }
  n177 = Merge Errors(w54, w49) -> (w26:errorcluster)
  n178 = disable-structure shown="Disabled" {
    frame Disabled {
      n179 = To Double Precision Float() -> (double precision float=w626:dbl)  [unwired: 1 in]
      n180 = To Double Precision Float() -> (double precision float=w627:dbl)  [unwired: 1 in]
      n181 = Subtract(x=w626, y=w627) -> (x-y=w625:dbl)
      n182 = Greater?(x=w625, y=10.0) -> (0:w624:bool)
      n183 = case shown="False" w624 {
        tunnel: [w628 w634] -> w623
        tunnel: [w629 w631] -> _
        tunnel: _ -> [w629 _]
        tunnel: [w628 w630] -> _
        frame False {
        }
        frame True {
          n184 = Get Date/Time In Seconds() -> (seconds since 1Jan1904=w631:timestamp)
          n185 = property on="Voltage 2" class="WFChart (strict)" props=["History Data", "XScale", "ScaleFit", "XScale", "Minimum", "XScale", "Maximum"](error in=w634, "History Data"=waveform(dbl)[][] []) -> (error out=w632:errorcluster)  [unwired: 4 in, 1 out]
          n186 = property on="Current 2" class="WFChart (strict)" props=["History Data", "XScale", "ScaleFit", "XScale", "Minimum", "XScale", "Maximum"](error in=w632) -> (error out=w630:errorcluster)  [unwired: 5 in, 1 out]
        }
      }
    }
    frame Enabled {
    }
  }
  n187 = Unbundle(w22) -> ("created path"=w5:path, "DCPowerInformation_byChannel"=w21:T10)  [unwired: 1 out]
  n188 = case shown="True" w10 {
    selector: w10 -> [w638 w670]
    tunnel: w26 -> [w637 w681]
    tunnel: [w637 w664] -> w25
    tunnel: [w643 w680] -> w20
    tunnel: w19 -> [w643 w679]
    tunnel: [w642 w678] -> w18
    tunnel: w17 -> [w642 w677]
    tunnel: [w641 w676] -> w16
    tunnel: w15 -> [w641 w675]
    tunnel: [w640 w674] -> w14
    tunnel: w13 -> [w640 w673]
    tunnel: [w639 w672] -> w12
    tunnel: w11 -> [w639 w671]
    tunnel: [w638 w670] -> w9
    tunnel: [string[][][] [] w669] -> w8
    tunnel: [string[][] [] ("DCPowerInfoArray") w659] -> w7
    tunnel: w5 -> [_ w662]
    frame False {
    }
    frame True {
      n189 = for {
        shift-right: [w683] -> w665
        shift-left: w681 -> [w695]
        tunnel: w671 -> [w686] mode=indexing
        shift-right: [w694] -> w680
        shift-left: w679 -> [w694]
        shift-right: [w693] -> w678
        shift-left: w677 -> [w693]
        shift-right: [w692] -> w676
        shift-left: w675 -> [w692]
        shift-right: [w691] -> w674
        shift-left: w673 -> [w691]
        shift-right: [w690] -> w672
        shift-left: w671 -> [w690]
        tunnel: [w682] -> w669 mode=indexing
        shift-right: [w688] -> w659
        shift-left: string[][] [] ("DCPowerInfoArray") -> [w689]
        # "This puts all the instruments together in one output"
        n190 = Unbundle(w686) -> ("instrument handle out"=w697:refnum<k15>, w696:string)  [unwired: 5 out]
        n191 = call <instrlib>:"niDCPower Abort With Channels.vi"("error in (no error)"=w695, "channel name"=w696, "instrument handle"=w697) -> ("error out"=w684:errorcluster)  [unwired: 7 in, 1 out]
        n192 = call "DCPower_ParameterCreation.vi"("error in"=w684, "Precision"="8", "DCPowerInformationByInstrument"=w686) -> ("error out"=w683:errorcluster, "DCPowerInfoArray"=w682:string[][])
        n193 = Insert Into Array(array=w689, index (col)=0 ("disabled index (col)"), new element=w682) -> (w688:string[][])  [unwired: 1 in]
      }
      n194 = Concatenate Strings("Channel Name " ("string")) -> (w654:string)
      n195 = Concatenate Strings("Voltage (V) " ("string")) -> (w656:string)
      n196 = Concatenate Strings("Measure Record delta Time (s) " ("string")) -> (w658:string)
      n197 = Concatenate Strings("Instrument Name " ("string")) -> (w653:string)
      n198 = Concatenate Strings("Instrument Channel Number " ("string")) -> (w655:string)
      n199 = Concatenate Strings("Current Limit (A) " ("string")) -> (w657:string)
      n200 = Build Array(w653, w654, w655, w656, w657, w658) -> (w646:string[])
      n201 = Insert Into Array(array=w659, index (col)=0 ("disabled index (col)"), new element=w646) -> (w645:string[][])  [unwired: 1 in]
      n202 = Build Path(base path=w662, name or relative path="DCPOW_Params.csv") -> (appended path=w663:path)
      n203 = call-poly <vilib>:"Write Delimited Spreadsheet.vi"("file path (dialog if empty)"=w663, "format (%s)"="%s" ("format (%.3f)"), "2D data"=w645, "error in (no error)"=w665, "transpose? (no:F)"=TRUE, "delimiter (\\t)"="," ("delimiter (\\t)")) -> ("error out"=w664:errorcluster)  [unwired: 8 in, 1 out]
    }
  }
  "DCPowerInformationClusterArray_Output" <- w12
  "VISAPowerInfoInputOutput" <- w14
  "Run Data SubPanel Output" <- w16
  "RF Block Parameters Output" <- w18
  "Oscilloscope Info Array Output" <- w20
  "Data Was Collected?" <- w9
  "Array" <- w8
  "DCPowerInfoArray" <- w7
  n204 = List Folder(path=w5, pattern="*.txt", error in=w25) -> (path out=w31:path, filenames=w30:string[], error out=w29:errorcluster)  [unwired: 1 in, 1 out]
  n205 = for {
    tunnel: [w698] -> w32
    tunnel: w31 -> [w698]
    tunnel: w30 -> [w700] mode=indexing
    shift-right: [w701] -> w28
    shift-left: w29 -> [w702]
    n206 = Build Path(base path=w698, name or relative path=w700) -> (appended path=w699:path)
    n207 = Delete(path (use dialog)=w699, error in=w702) -> (error out=w701:errorcluster)  [unwired: 3 in, 2 out]
  }
  n208 = Strip Path(path=w32) -> (name=w36:string)  [unwired: 1 out]
  n209 = Concatenate Strings(w36, "_DCPOWER_COPYFOLDER" ("name or relative path")) -> (w34:string)
  n210 = Build Path(base path=w32, name or relative path=w34) -> (appended path=w44:path)
  n211 = Create Folder(path (use dialog)=w44, error in=w28) -> (created path=w39:path, error out=w42:errorcluster)  [unwired: 1 in, 1 out]
  n212 = List Folder(path=w32, error in=w42) -> (path out=w41:path, filenames=w40:string[], error out=w38:errorcluster)  [unwired: 2 in, 1 out]
  n213 = for {
    tunnel: w41 -> [w708]
    tunnel: w40 -> [w707] mode=indexing
    tunnel: w39 -> [w703]
    shift-right: [w710] -> w43
    shift-left: w38 -> [w704]
    tunnel: [w703] -> w37
    n214 = Build Path(base path=w708, name or relative path=w707) -> (appended path=w705:path)
    n215 = Build Path(base path=w703, name or relative path=w707) -> (appended path=w706:path)
    n216 = Copy(8:w704, 9:TRUE ("overwrite (F)"), 10:w706, 11:w705) -> (0:w710:errorcluster)  [unwired: 1 in, 2 out]
  }
  n217 = disable-structure shown="Enabled" {
    disable-tunnel: [w719 w720] -> w48
    disable-tunnel: w21 -> [w718 _]
    disable-tunnel: w43 -> [w716 w720]
    disable-tunnel: w37 -> [w715 _]
    frame Disabled {
      n218 = Two Button Dialog(message="Create CSVs for every channel now? (Processing Time will take longer)", 1:"NO" ("F button name (\"Cancel\")"), 2:"YES" ("T button name (\"OK\")")) -> (T button?=w711:bool)
      n219 = call "ReadDataFile_V1.vi"("error in (no error)"=w716, "Create CSV files?"=w711, "Channel Names Array"=w718, "DataFolder Path"=w715) -> ("error out"=w719:errorcluster, "Voltage Measurements"=w717:cluster{dbl[], dbl[]}[])  [unwired: 5 in, 1 out]
    }
    frame Enabled {
    }
  }
  "error out" <- w48
